vi "Selected Index Write.vi"(4 "error in (no error)":errorcluster, 5 "Value":i32[](array[numeric]), 6 "Container State":T2, 7 "Display State In":T1) -> (0 "error out":errorcluster, 3 "Display State Out":T1)   [LabVIEW 2014, in "ListBox XControl.xctl"]
uses:
  ListBox XControl.xctl
  <vilib>/_xctls/Container State.ctl
  State ListBox.ctl
  <vilib>/_xctls/XControlSupport.lvlib
panel:
  # "Replace the Value Control below with a Control of desired type.\nDo not remove this Control or the others from the connector pane.\nDo not change the connector pane pattern.\nThe Value control should always be the third terminal from top on the input side in the connector pane."
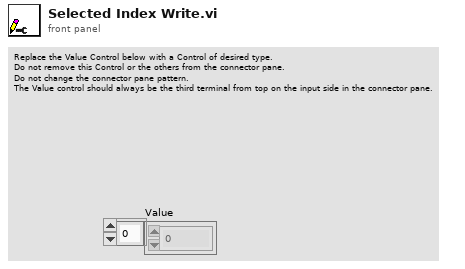
[diagram p1: front panel]
types:
  T1 = typedef "ListBox XControl.xctl/State ListBox.ctl" = cluster{"ItemNames[]":string[], "Listbox Ref":refnum<vi>, "Select All By Default":bool}
  T2 = typedef "XControlSupport.lvlib/Container State.ctl" = cluster{"Indicator?":bool, "Run Mode?":bool, " Refnum":refnum<vi>}
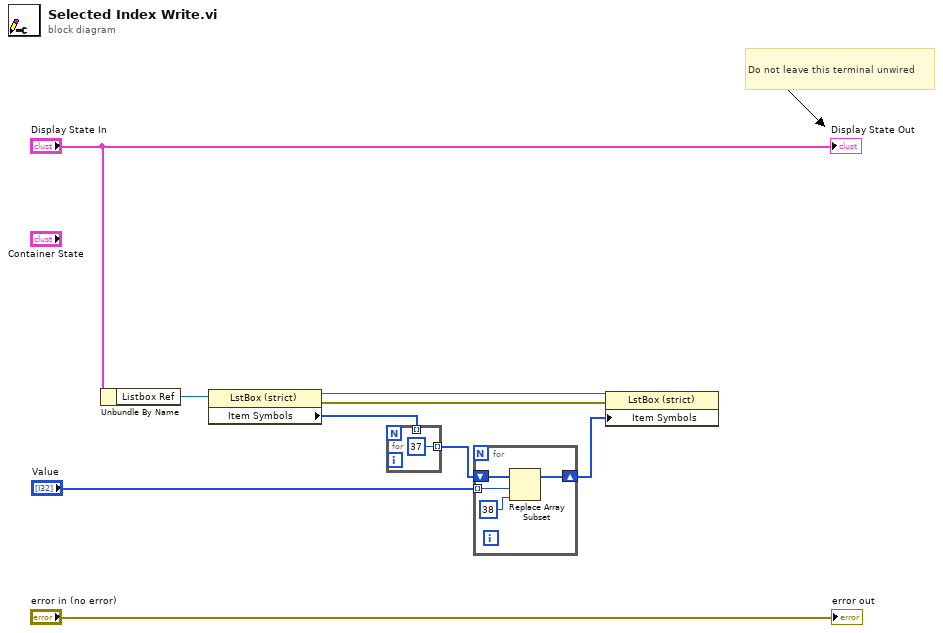
[diagram p0: block diagram]
diagram:
  # "Do not leave this terminal unwired"
  n1 = Unbundle By Name("Display State In") -> ("Listbox Ref"=w8:refnum<vi>)
  n2 = property class="LstBox (strict)"(reference=w8) -> (reference out=w6:refnum<vi>, error out=w4:errorcluster, "Item Symbols"=w2:i32[])  [unwired: 1 in]
  n3 = for {
    tunnel: w2 -> [_] mode=indexing
    tunnel: [37 ("new element/subarray")] -> w1 mode=indexing
  }
  n4 = for {
    shift-right: [w13] -> w5
    shift-left: w1 -> [w14]
    tunnel: "Value" -> [w12] mode=indexing
    n5 = Replace Array Subset(array=w14, new element=38 ("new element/subarray"), index=w12) -> (w13:i32[])
  }
  n6 = property class="LstBox (strict)"(reference=w6, error in=w4, "Item Symbols"=w5) -> ()  [unwired: 2 out]
  "error out" <- "error in (no error)"
  "Display State Out" <- "Display State In"
